vi "Append Delays to Waveform.vi"(9 "Post Delay (s)":dbl=0.001 format="%#_6p", 10 "Pre Delay (s)":dbl=0.001 format="%#_6p", 11 "Input Waveform":waveform(dbl)) -> (3 "Output Waveform":waveform(dbl)(graph))   [LabVIEW 2025]
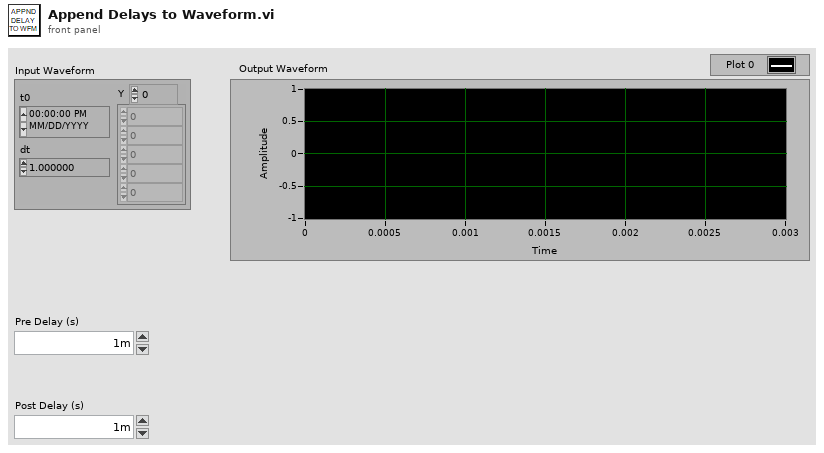
[diagram p1: front panel]
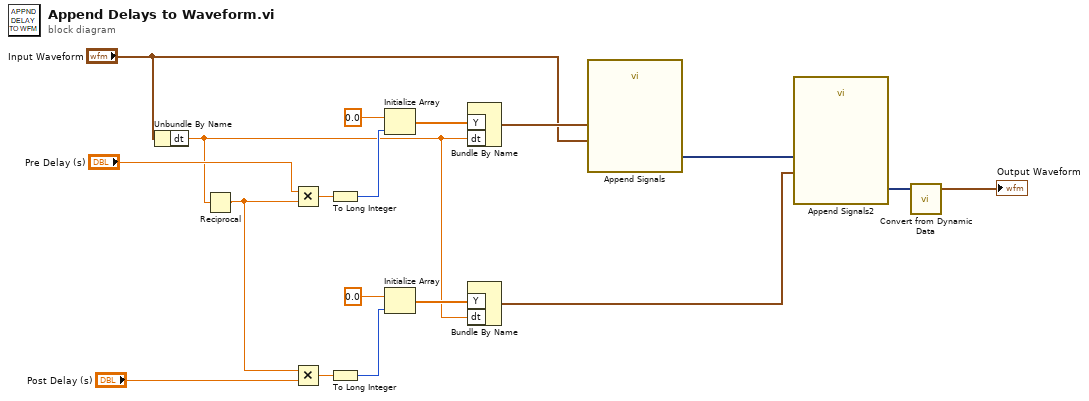
[diagram p0: block diagram]
diagram:
  n1 = Unbundle By Name("Input Waveform") -> ("dt"=w2:dbl)
  n2 = Reciprocal(x=w2) -> (1/x=w3:dbl)
  n3 = Multiply(x="Pre Delay (s)", y=w3) -> (x*y=w18:dbl)
  n4 = Multiply(x=w3, y="Post Delay (s)") -> (x*y=w10:dbl)
  n5 = To Long Integer(number=w18) -> (32bit integer=w16:i32)
  n6 = To Long Integer(number=w10) -> (32bit integer=w9:i32)
  n7 = Initialize Array(0.0 ("DC Value"), w16) -> (w17:dbl[])
  n8 = Initialize Array(0.0 ("DC Value"), w9) -> (w12:dbl[])
  n9 = Bundle By Name("Y"=w17, "dt"=w2) -> (w8:waveform(dbl))  [unwired: 1 in]
  n10 = Bundle By Name("Y"=w12, "dt"=w2) -> (w6:waveform(dbl))  [unwired: 1 in]
  n11 = call "Append Signals"("Input Signal B"="Input Waveform", "Input Signal A"=w8) -> ("Appended Signals"=w7:dynamicdata)  [unwired: 8 in, 1 out]
  n12 = call "Append Signals2"("Input Signal B"=w6, "Input Signal A"=w7) -> ("Appended Signals"=w5:dynamicdata)  [unwired: 8 in, 1 out]
  n13 = call "Convert from Dynamic Data"("Dynamic Data Type"=w5) -> ("Waveform"=→"Output Waveform":waveform(dbl))  [unwired: 3 in]
